vi "subDFD_Build Filter Bank Tree.vi"(8 "error in (no error)":errorcluster, 9 "bank to append":T1 {"mFBank_SynthesisFilters"."mMRate_SumWl" min=1 max=32 step=1; "mFBank_SynthesisFilters"."mMRate_InputIwl" min=1 max=32 step=1; "mFBank_SynthesisFilters"."mMRate_GainWl" min=1 max=32 step=1; "mFBank_SynthesisFilters"."mMRate_OutputWl" min=1 max=32 step=1; "mFBank_SynthesisFilters"."mMRate_InputWl" min=1 max=32 step=1; "mFBank_SynthesisFilters"."mMRate_CoefWl" min=1 max=32 step=1; "mFBank_SynthesisFilters"."mMRate_Mode" items=["Default"=-1, "No Rate Change"=0, "Interpolation"=1, "Decimation"=2, "Interpolated"=3, "Rational"=4]; "mFBank_AnalysisFilters"."mMRate_SumWl" min=1 max=32 step=1; "mFBank_AnalysisFilters"."mMRate_InputIwl" min=1 max=32 step=1; "mFBank_AnalysisFilters"."mMRate_GainWl" min=1 max=32 step=1; "mFBank_AnalysisFilters"."mMRate_OutputWl" min=1 max=32 step=1; "mFBank_AnalysisFilters"."mMRate_InputWl" min=1 max=32 step=1; "mFBank_AnalysisFilters"."mMRate_CoefWl" min=1 max=32 step=1; "mFBank_AnalysisFilters"."mMRate_Mode" items=["Default"=-1, "No Rate Change"=0, "Interpolation"=1, "Decimation"=2, "Interpolated"=3, "Rational"=4]; "mFBank_Type" items=["Uniform", "Non-Uniform"]}, 10 "branch index":i32, 11 "tree in":T1={"mFBank_AnalysisFilters"=[], "mFBank_SynthesisFilters"=[], "mFBank_#Bands"=0, "mFBank_ProcMethod"=enum."General", "mFBank_Coeffs"=[], "mFBank_Gain"=1.0, "mFBank_Delay"=0, "mFBank_Type"=0} {"mFBank_SynthesisFilters"."mMRate_SumWl" min=1 max=32 step=1; "mFBank_SynthesisFilters"."mMRate_InputIwl" min=1 max=32 step=1; "mFBank_SynthesisFilters"."mMRate_GainWl" min=1 max=32 step=1; "mFBank_SynthesisFilters"."mMRate_OutputWl" min=1 max=32 step=1; "mFBank_SynthesisFilters"."mMRate_InputWl" min=1 max=32 step=1; "mFBank_SynthesisFilters"."mMRate_CoefWl" min=1 max=32 step=1; "mFBank_SynthesisFilters"."mMRate_Mode" items=["Default"=-1, "No Rate Change"=0, "Interpolation"=1, "Decimation"=2, "Interpolated"=3, "Rational"=4]; "mFBank_AnalysisFilters"."mMRate_SumWl" min=1 max=32 step=1; "mFBank_AnalysisFilters"."mMRate_InputIwl" min=1 max=32 step=1; "mFBank_AnalysisFilters"."mMRate_GainWl" min=1 max=32 step=1; "mFBank_AnalysisFilters"."mMRate_OutputWl" min=1 max=32 step=1; "mFBank_AnalysisFilters"."mMRate_InputWl" min=1 max=32 step=1; "mFBank_AnalysisFilters"."mMRate_CoefWl" min=1 max=32 step=1; "mFBank_AnalysisFilters"."mMRate_Mode" items=["Default"=-1, "No Rate Change"=0, "Interpolation"=1, "Decimation"=2, "Interpolated"=3, "Rational"=4]; "mFBank_Type" items=["Uniform", "Non-Uniform"]}) -> (0 "error out":errorcluster, 3 "tree out":T1={"mFBank_AnalysisFilters"=[], "mFBank_SynthesisFilters"=[], "mFBank_#Bands"=0, "mFBank_ProcMethod"=enum."General", "mFBank_Coeffs"=[], "mFBank_Gain"=1.0, "mFBank_Delay"=0, "mFBank_Type"=0} {"mFBank_SynthesisFilters"."mMRate_SumWl" min=1 max=32 step=1; "mFBank_SynthesisFilters"."mMRate_InputIwl" min=1 max=32 step=1; "mFBank_SynthesisFilters"."mMRate_GainWl" min=1 max=32 step=1; "mFBank_SynthesisFilters"."mMRate_OutputWl" min=1 max=32 step=1; "mFBank_SynthesisFilters"."mMRate_InputWl" min=1 max=32 step=1; "mFBank_SynthesisFilters"."mMRate_CoefWl" min=1 max=32 step=1; "mFBank_SynthesisFilters"."mMRate_Mode" items=["Default"=-1, "No Rate Change"=0, "Interpolation"=1, "Decimation"=2, "Interpolated"=3, "Rational"=4]; "mFBank_AnalysisFilters"."mMRate_SumWl" min=1 max=32 step=1; "mFBank_AnalysisFilters"."mMRate_InputIwl" min=1 max=32 step=1; "mFBank_AnalysisFilters"."mMRate_GainWl" min=1 max=32 step=1; "mFBank_AnalysisFilters"."mMRate_OutputWl" min=1 max=32 step=1; "mFBank_AnalysisFilters"."mMRate_InputWl" min=1 max=32 step=1; "mFBank_AnalysisFilters"."mMRate_CoefWl" min=1 max=32 step=1; "mFBank_AnalysisFilters"."mMRate_Mode" items=["Default"=-1, "No Rate Change"=0, "Interpolation"=1, "Decimation"=2, "Interpolated"=3, "Rational"=4]; "mFBank_Type" items=["Uniform", "Non-Uniform"]})   [LabVIEW 2023]
uses:
  <vilib>/addons/Digital Filter Design/FilterBank.llb/Object/DFD Filter Bank Obj.ctl
  <vilib>/addons/Digital Filter Design/_Objects.llb/DFD Multirate Filter Obj.ctl
  <vilib>/addons/Digital Filter Design/_Objects.llb/DFD Multirate Mode.ctl
  <vilib>/addons/Digital Filter Design/_Objects.llb/DFD Coef Norm Type.ctl
  <vilib>/addons/Digital Filter Design/_Objects.llb/DFD Round-off Mode.ctl
  <vilib>/addons/Digital Filter Design/_Objects.llb/DFD FXP MRate Multiply Mode.ctl
  <vilib>/addons/Digital Filter Design/FilterBank.llb/Object/DFD Filter Bank Processing Method.ctl
  <vilib>/addons/Digital Filter Design/FilterBank.llb/Object/DFD Filter Bank Type.ctl
  <vilib>/addons/Digital Filter Design/NI_DigFilter_FilterBank.lvlib
  <vilib>/addons/Digital Filter Design/NI_DigFilterLicensed.lvlib
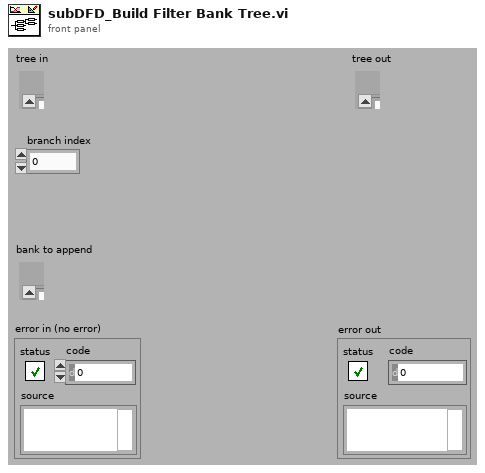
[diagram p1: front panel]
types:
  T1 = typedef "NI_DigFilter_FilterBank.lvlib/DFD Filter Bank Obj.ctl" = cluster{"mFBank_AnalysisFilters":T2[], "mFBank_SynthesisFilters":T2[], "mFBank_#Bands":i32, "mFBank_ProcMethod":T7, "mFBank_Coeffs":dbl[], "mFBank_Gain":dbl, "mFBank_Delay":i32, "mFBank_Type":T8}
  T2 = typedef "NI_DigFilterLicensed.lvlib/DFD Multirate Filter Obj.ctl" = cluster{"mMRate_Structure":enum16{"CIC", "FIR", "IIR", "Lattice"}, "mMRate_Mode":T3, "mMRate_Factor":i32, "mMRate_FIRParams":cluster{"mMRate_FIR_H":dbl[], "mMRate_FIR_IsNyquist?":bool, "mMRate_FIR_IsSymmetric?":bool}, "mMRate_CICParams":cluster{"mMRate_CIC_#Stage":i32, "mMRate_CIC_Lag":i32, "mMRate_CIC_Type":enum16{"Lowpass", "Highpass"}}, "mMRate_Order":i32, "mMRate_Version":string, "mMRate_Comments":string, "mMRate_RationalFactor":cluster{"mMRate_L":i32, "mMRate_M":i32}, "mMRate_Fs":dbl, "mMRate_Quantized?":bool, "mMRate_QFilterGain":dbl, "mMRate_CoefWl":i16, "mMRate_Scaling":cluster{"mMRate_ScaleByPowerOf2?":bool, "mMRate_ScaleType":T4}, "mMRate_InputWl":i16, "mMRate_OutputWl":i16, "mMRate_OutputMode":T5, "mMRate_MultMode":T6, "mMRate_BitPruning":bool, "mMRate_GainWl":i16, "mMRate_OutputFwl":i16, "mMRate_SumIwl":i16, "mMRate_InputIwl ":i16, "mMRate_SumWl":i16, "mMRate_CoefIwl":i16}
  T3 = typedef "NI_DigFilterLicensed.lvlib/DFD Multirate Mode.ctl" = i16
  T4 = typedef "NI_DigFilterLicensed.lvlib/DFD Coef Norm Type.ctl" = enum16{"No Norm", "Time Domain 1-Norm", "Time Domain 2-Norm", "Time Domain Inf-Norm"}
  T5 = typedef "NI_DigFilterLicensed.lvlib/DFD Round-off Mode.ctl" = enum16{"Nearest", "Truncation"}
  T6 = typedef "NI_DigFilterLicensed.lvlib/DFD FXP MRate Multiply Mode.ctl" = enum16{"Truncated", "Full"}
  T7 = typedef "NI_DigFilter_FilterBank.lvlib/DFD Filter Bank Processing Method.ctl" = enum16{"General", "2-Band QMF Lattice", "Cosine-Modulated"}
  T8 = typedef "NI_DigFilter_FilterBank.lvlib/DFD Filter Bank Type.ctl" = u16
  T9 = typedef "NI_DigFilter_FilterBank.lvlib/DFD Bank Obj.ctl" = cluster{"mBank_Filters":T2[], " mBank_#Bands":i32, "mBank_ProcMethod":T7, "mBank_Coeffs":dbl[], "mBank_Gain":dbl, "mBank_Type":T8}
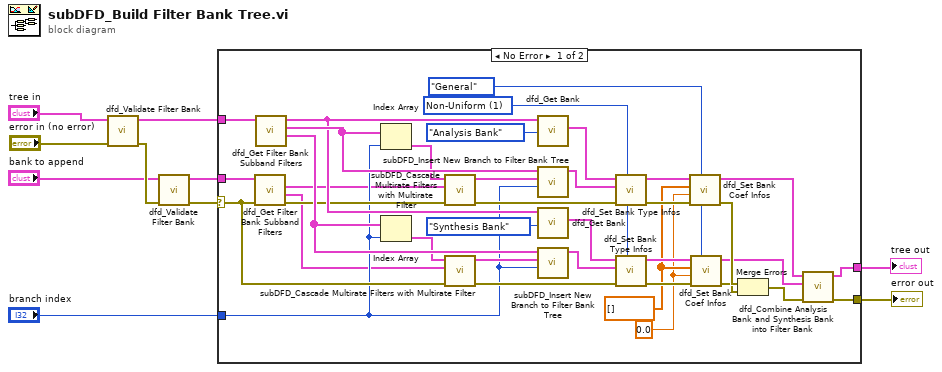
[diagram p0: block diagram]
diagram:
  n1 = call <vilib>:"dfd_Validate Filter Bank.vi"("error in (no error)"="error in (no error)", "filter banks in"="tree in") -> ("error out"=w5:errorcluster, "filter bank out"=w1:T1)  [unwired: 7 in, 1 out]
  n2 = call <vilib>:"dfd_Validate Filter Bank.vi"("error in (no error)"=w5, "filter banks in"="bank to append") -> ("error out"=w4:errorcluster, "filter bank out"=w2:T1)  [unwired: 7 in, 1 out]
  n3 = case shown="No Error" w4 {
    selector: w4 -> [w25 w47]
    tunnel: w2 -> [w46 _]
    tunnel: w1 -> [w15 _]
    tunnel: [w12 _] -> w8
    tunnel: "branch index" -> [w16 _]
    tunnel: [w11 w47] -> w9
    frame No Error {
      w26 = DFD_Filter_Bank_Processing_Method."General" ("type")
      w27 = 0.0 ("gain")
      w28 = dbl[] [] ("coefficients")
      w33 = T8 1 items=["Uniform", "Non-Uniform"] ("bank type")
      n4 = call <vilib>:"dfd_Get Filter Bank Subband Filters.vi"("filter bank in"=w46) -> ("synthesis filters"=w13:T2[], "analysis filters"=w14:T2[])  [unwired: 7 in, 2 out]
      n5 = call <vilib>:"dfd_Get Filter Bank Subband Filters.vi"("filter bank in"=w15) -> ("synthesis filters"=w35:T2[], "analysis filters"=w42:T2[], "filter bank out"=w34:T1)  [unwired: 7 in, 1 out]
      n6 = Index Array(array=w42, index=w16) -> (element=w40:T2)
      n7 = Index Array(array=w35, index=w16) -> (element=w17:T2)
      n8 = call "subDFD_Cascade Multirate Filters with Multirate Filter.vi"("error in (no error)"=w25, "multirate filters"=w14, "multirate filter"=w40) -> ("error out"=w24:errorcluster, "cascaded filters"=w43:T2[])  [unwired: 7 in]
      n9 = call "subDFD_Cascade Multirate Filters with Multirate Filter.vi"("error in (no error)"=w25, "multirate filters"=w13, "multirate filter"=w17) -> ("error out"=w23:errorcluster, "cascaded filters"=w38:T2[])  [unwired: 7 in]
      n10 = call <vilib>:"dfd_Get Bank.vi"("bank type"=enum16{"Analysis Bank", "Synthesis Bank"}."Analysis Bank", "filter bank"=w34) -> ("bank"=w45:T9)  [unwired: 7 in, 2 out]
      n11 = call "subDFD_Insert New Branch to Filter Bank Tree.vi"("branch index"=w16, "cascaded filters"=w43, "multirate filters"=w42) -> ("new multirate filters"=w41:T2[])  [unwired: 8 in]
      n12 = call <vilib>:"dfd_Get Bank.vi"("bank type"=enum16{"Analysis Bank", "Synthesis Bank"}."Synthesis Bank", "filter bank"=w34) -> ("bank"=w36:T9)  [unwired: 7 in, 2 out]
      n13 = call "subDFD_Insert New Branch to Filter Bank Tree.vi"("branch index"=w16, "cascaded filters"=w38, "multirate filters"=w35) -> ("new multirate filters"=w39:T2[])  [unwired: 8 in]
      n14 = call <vilib>:"dfd_Set Bank Type Infos.vi"("filter bank type"=w33, "error in (no error)"=w24, "subband filters"=w41, "bank in"=w45) -> ("error out"=w31:errorcluster, "bank out"=w32:T9)  [unwired: 2 in, 4 out]
      n15 = call <vilib>:"dfd_Set Bank Type Infos.vi"("filter bank type"=w33, "error in (no error)"=w23, "subband filters"=w39, "bank in"=w36) -> ("error out"=w29:errorcluster, "bank out"=w30:T9)  [unwired: 2 in, 4 out]
      n16 = call <vilib>:"dfd_Set Bank Coef Infos.vi"("type"=w26, "error in (no error)"=w31, "gain"=w27, "coefficients"=w28, "bank in"=w32) -> ("error out"=w22:errorcluster, "bank out"=w19:T9)  [unwired: 5 in]
      n17 = call <vilib>:"dfd_Set Bank Coef Infos.vi"("type"=w26, "error in (no error)"=w29, "gain"=w27, "coefficients"=w28, "bank in"=w30) -> ("error out"=w21:errorcluster, "bank out"=w18:T9)  [unwired: 5 in]
      n18 = Merge Errors(w22, w21) -> (w20:errorcluster)
      n19 = call <vilib>:"dfd_Combine Analysis Bank and Synthesis Bank into Filter Bank.vi"("error in (no error)"=w20, "synthesis bank"=w18, "analysis bank"=w19) -> ("error out"=w11:errorcluster, "filter bank out"=w12:T1)  [unwired: 7 in]
    }
    frame Error {
    }
  }
  "tree out" <- w8
  "error out" <- w9
